vi "datain.vi"(11 "output":dbl) -> ()   [LabVIEW 2017, in "HapticSTM.lvlib"]
doc: "extern \"C\" __declspec(dllexport) void datain(double output);"
uses:
  <userlib>/HapticSTM/Feedbackless - Testdata/Project/feedbackless.lvproj/HapticSTM.lvlib
  <userlib>/HapticSTM/HapticSTM.dll
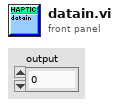
[diagram p1: front panel]
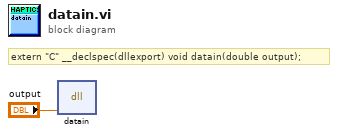
[diagram p0: block diagram]
diagram:
  # "extern \"C\" __declspec(dllexport) void datain(double output);"
  n1 = dll-call lib="C:/Program Files/National Instruments/LabVIEW 2019/user.lib/HapticSTM/HapticSTM.*" fn="datain"("output"="output") -> ()  [unwired: 5 in, 2 out]
